vi "Record Minimum Distance Of Adjascents.vi"(8 "Column In":i32, 9 "Row In":i32, 10 "Minimum Distance Matrix In":u32[][](array[numeric]), 11 "Data Matrix":u8[][](array[numeric])) -> (0 "Columns Out":i32[](array[numeric]), 1 "Rows Out":i32[](array[numeric]), 2 "Minimum Distance Matrix Out":u32[][](array[numeric]))   [LabVIEW 2019, in "Day 15.lvlib"]
uses:
  Day 15.lvlib
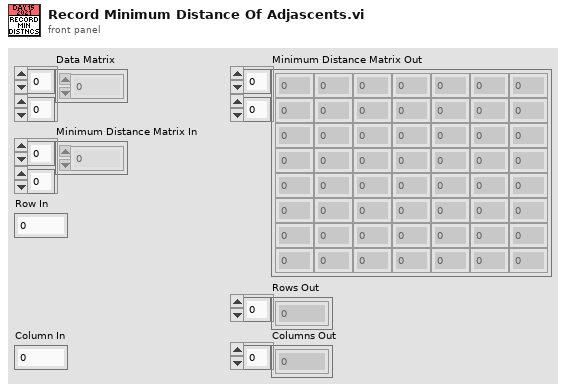
[diagram p1: front panel]
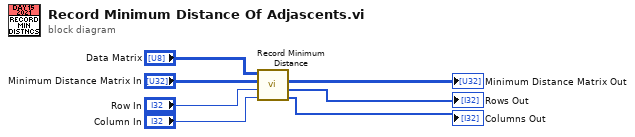
[diagram p0: block diagram]
diagram:
  n1 = call "Record Minimum Distance.vi"("Column"="Column In", "Row"="Row In", "Minimum Distance Matrix"="Minimum Distance Matrix In", "Main Matrix"="Data Matrix") -> ("Columns Out"=→"Columns Out":i32[], "Rows Out"=→"Rows Out":i32[], "Minimum Distance Matrix Out"=→"Minimum Distance Matrix Out":u32[][])  [unwired: 5 in]
